vi "gentec-M-Link.Set Block Signal.vi"(0 "VISA resource In":refnum<visa-resource-name>, 2 "Block Signal":bool, 5 "error in (no error)":errorcluster) -> (14 "VISA resource Out":refnum<visa-resource-name>, 19 "error out":errorcluster)   [LabVIEW 2014, in "gentec-M-Link - Driver.lvlib"]
doc: "Data to write: sql0 or sql1\n\nCommand only. This command blocks the signal to the instrument. It is used to synchronize two instruments in dual channel usage.\n\nsql1 (true) will block the signal and stop triggering.\nsql0 (false) will unblock the signal and start triggering.\n\nThis allows two instruments in energy mode to start triggering on the same pulse."
uses:
  gentec-M-Link - Driver.lvlib
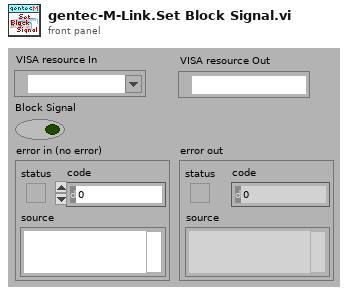
[diagram p1: front panel]
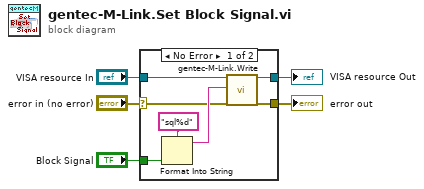
[diagram p0: block diagram]
diagram:
  n1 = case shown="No Error" "error in (no error)" {
    selector: "error in (no error)" -> [w10 w14]
    tunnel: [w6 w14] -> w4
    tunnel: "VISA resource In" -> [w9 w13]
    tunnel: [w7 w13] -> w2
    tunnel: "Block Signal" -> [w8 _]
    frame No Error {
      n2 = Format Into String(format string="sql%d", w8) -> (resulting string=w11:string)  [unwired: 2 in, 1 out]
      n3 = call "gentec-M-Link.Write.vi"("VISA resource (In)"=w9, "Data To Write"=w11, "error in (no error)"=w10) -> ("VISA resource (Out)"=w7:refnum<visa-resource-name>, "error out"=w6:errorcluster)  [unwired: 14 in, 1 out]
    }
    frame Error {
    }
  }
  "error out" <- w4
  "VISA resource Out" <- w2
